vi "IsTheDUTStillConnected.vi"(11 "EBLer":dbl[][](array[numeric])) -> (2 "Connected":bool, 3 "Reliability Indicator":dbl)   [LabVIEW 2013]
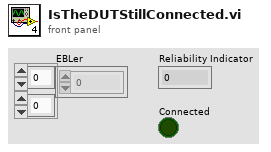
[diagram p1: front panel]
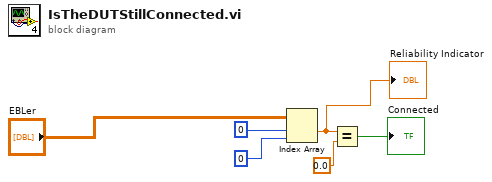
[diagram p0: block diagram]
diagram:
  n1 = Index Array(array="EBLer", index (row)=0 ("index"), index (col)=0 ("disabled index (col)")) -> (element=w6:dbl)
  "Reliability Indicator" <- w6
  n2 = Equal?(x=w6, y=0.0) -> (x = y?=→"Connected":bool)
